vi "OEE_destroy_queues.vi"(8 "error_in":errorcluster, 11 "all_config_info":T1={"main_ini_file"={"SQL Driver"="", "SQL Server"="", "SQL Database"="", "SQL UID"="", "Reference table"="", "Reference history"="", "Archivisation CFG table"="", "Archivisation CFG history"="", "User table"="", "User history"="", "Default reference"="", "Update pulse[ms]"=0, "default language"="", "SCREEN 1 Left"=0, "SCREEN 1 Top"=10, "SCREEN 1 Width"=0, "SCREEN 1 Height"=0, "SCREEN 2 Left"=0, "SCREEN 2 Top"=0, "SCREEN 2 Width"=0, "SCREEN 2 Height"=10}, "SQL Password"="", "queue_refnums"={"MAIN_queue"=refnum, "SCREEN_1_queue"=refnum, "SCREEN_2_queue"=refnum, "PULSE_queue"=refnum, "GRAPH_TOGGLE_queue"=refnum}}) -> (0 "error_out":errorcluster)   [LabVIEW 2019]
uses:
  ini/typedef/OEE_all_config_info.ctl
  ini/typedef/OEE_main_ini_file.ctl
  typedef/OEE_queue_refnums.ctl
  typedef/OEE_MAIN_queue_element.ctl
  MAIN/OEE_MAIN_sequence_state.ctl
  typedef/OEE_SCREEN_1_queue_element.ctl
  SCREEN_1/OEE_SCREEN_1_sequence_state.ctl
  typedef/OEE_SCREEN_2_queue_element.ctl
  SCREEN_2/OEE_SCREEN_2_sequence_state.ctl
  typedef/OEE_PULSE_queue_element.ctl
  PULSE/OEE_PULSE_sequence_state.ctl
  typedef/OEE_GRAPH_TOGGLE_TIMER_queue_element.ctl
  SCREEN_2/GRAPH_TOGGLE_TIMER/OEE_GRAPH_TOGGLE_TIMER_sequence_state.ctl
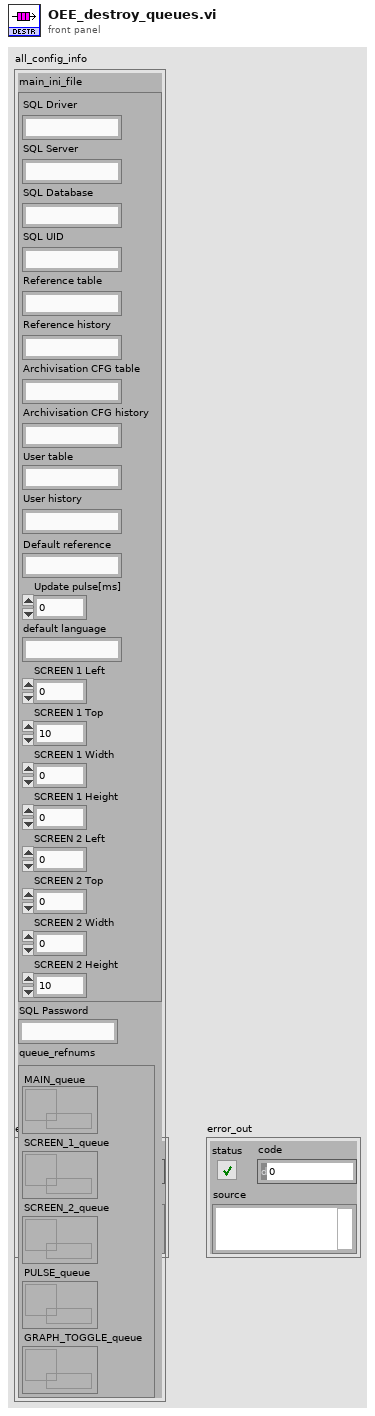
[diagram p1: front panel]
types:
  T1 = typedef "OEE_all_config_info.ctl" = cluster{"main_ini_file":T2, "SQL Password":string, "queue_refnums":T3}
  T2 = typedef "OEE_main_ini_file.ctl" = cluster{"SQL Driver":string, "SQL Server":string, "SQL Database":string, "SQL UID":string, "Reference table":string, "Reference history":string, "Archivisation CFG table":string, "Archivisation CFG history":string, "User table":string, "User history":string, "Default reference":string, "Update pulse[ms]":i32, "default language":string, "SCREEN 1 Left":i16, "SCREEN 1 Top":i16, "SCREEN 1 Width":i16, "SCREEN 1 Height":i16, "SCREEN 2 Left":i16, "SCREEN 2 Top":i16, "SCREEN 2 Width":i16, "SCREEN 2 Height":i16}
  T3 = typedef "OEE_queue_refnums.ctl" = cluster{"MAIN_queue":refnum<queue>, "SCREEN_1_queue":refnum<queue>, "SCREEN_2_queue":refnum<queue>, "PULSE_queue":refnum<queue>, "GRAPH_TOGGLE_queue":refnum<queue>}
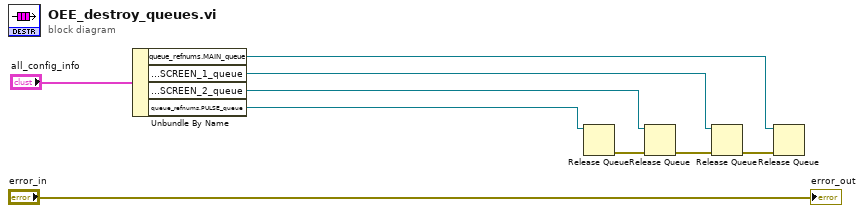
[diagram p0: block diagram]
diagram:
  n1 = Unbundle By Name("all_config_info") -> ("queue_refnums.MAIN_queue"=w1:refnum<queue>, "queue_refnums.SCREEN_1_queue"=w7:refnum<queue>, "queue_refnums.SCREEN_2_queue"=w5:refnum<queue>, "queue_refnums.PULSE_queue"=w2:refnum<queue>)
  n2 = Release Queue(queue=w2) -> (error out=w4:errorcluster)  [unwired: 2 in, 2 out]
  n3 = Release Queue(queue=w5, error in (no error)=w4) -> (error out=w6:errorcluster)  [unwired: 1 in, 2 out]
  n4 = Release Queue(queue=w7, error in (no error)=w6) -> (error out=w3:errorcluster)  [unwired: 1 in, 2 out]
  n5 = Release Queue(queue=w1, error in (no error)=w3) -> ()  [unwired: 1 in, 3 out]
  "error_out" <- "error_in"
